vi "WristNetwork_ReadSlow.vi"(8 "error in (no error)":errorcluster) -> (0 "error out":errorcluster)   [LabVIEW 2023]
uses:
  WristGlobal.vi
  <vilib>/Rock Robotics/Network Tables/NT Read Number.vi
  <vilib>/Rock Robotics/Network Tables/NT Read Boolean.vi
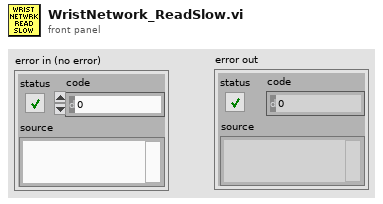
[diagram p1: front panel]
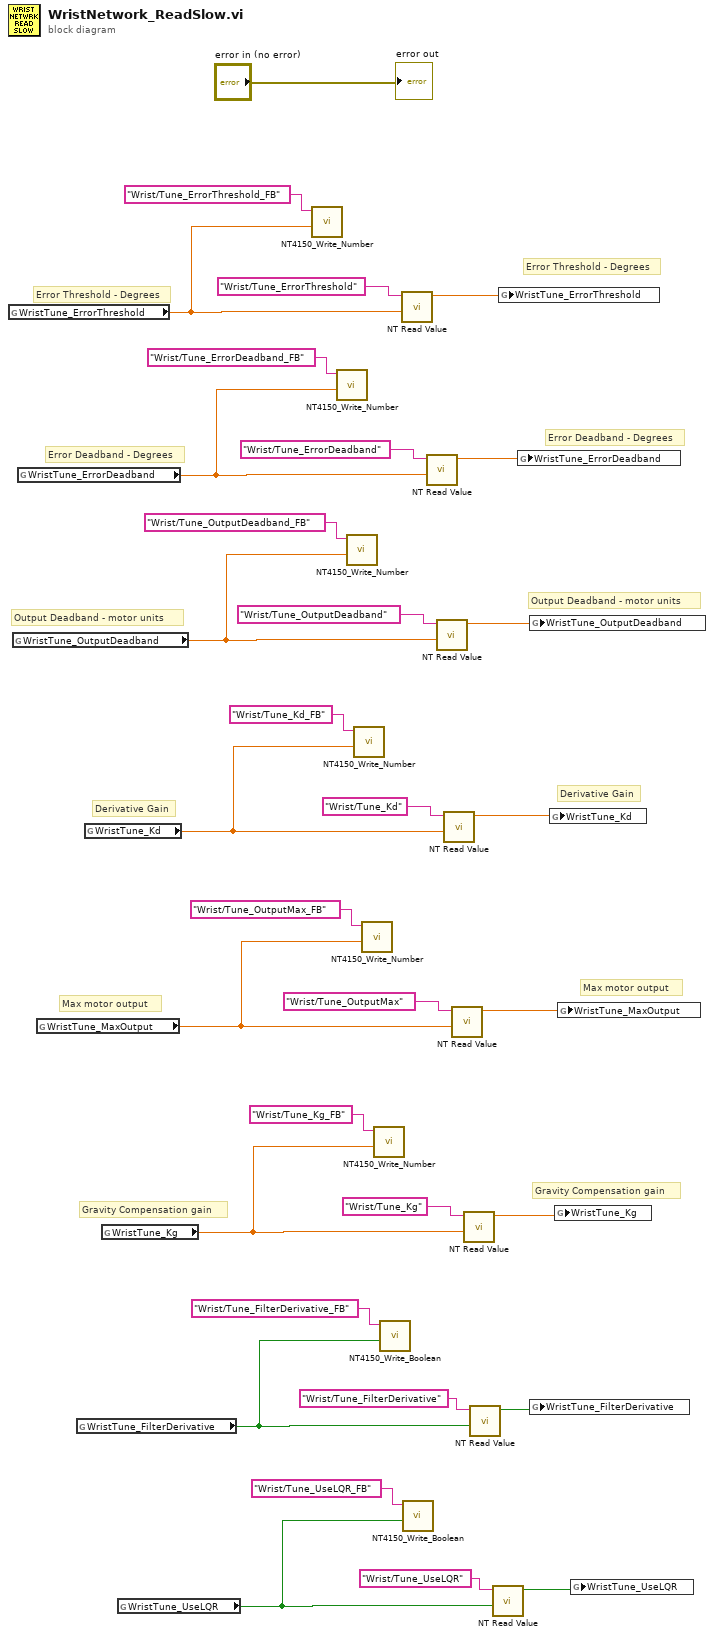
[diagram p0: block diagram]
diagram:
  # "Gravity Compensation gain"
  # "Max motor output"
  # "Derivative Gain"
  # "Output Deadband - motor units"
  # "Error Deadband - Degrees"
  # "Error Threshold - Degrees"
  # "Gravity Compensation gain"
  # "Max motor output"
  # "Derivative Gain"
  # "Output Deadband - motor units"
  # "Error Deadband - Degrees"
  # "Error Threshold - Degrees"
  n1 = global read "WristGlobal.vi" "WristTune_ErrorThreshold"() -> (w30:dbl)
  n2 = global read "WristGlobal.vi" "WristTune_OutputDeadband"() -> (w16:dbl)
  n3 = global read "WristGlobal.vi" "WristTune_ErrorDeadband"() -> (w26:dbl)
  n4 = global read "WristGlobal.vi" "WristTune_MaxOutput"() -> (w12:dbl)
  n5 = global read "WristGlobal.vi" "WristTune_FilterDerivative"() -> (w6:bool)
  n6 = global read "WristGlobal.vi" "WristTune_Kd"() -> (w14:dbl)
  n7 = global read "WristGlobal.vi" "WristTune_Kg"() -> (w10:dbl)
  n8 = global read "WristGlobal.vi" "WristTune_UseLQR"() -> (w2:bool)
  n9 = call "NT4150_Write_Number.vi"("value"=w30, "name"="Wrist/Tune_ErrorThreshold_FB") -> ()  [unwired: 9 in, 1 out]
  n10 = call "NT4150_Write_Number.vi"("value"=w26, "name"="Wrist/Tune_ErrorDeadband_FB") -> ()  [unwired: 9 in, 1 out]
  n11 = call "NT4150_Write_Number.vi"("value"=w16, "name"="Wrist/Tune_OutputDeadband_FB") -> ()  [unwired: 9 in, 1 out]
  n12 = call "NT4150_Write_Number.vi"("value"=w14, "name"="Wrist/Tune_Kd_FB") -> ()  [unwired: 9 in, 1 out]
  n13 = call "NT4150_Write_Number.vi"("value"=w12, "name"="Wrist/Tune_OutputMax_FB") -> ()  [unwired: 9 in, 1 out]
  n14 = call "NT4150_Write_Number.vi"("value"=w10, "name"="Wrist/Tune_Kg_FB") -> ()  [unwired: 9 in, 1 out]
  n15 = call "NT4150_Write_Boolean.vi"("value"=w6, "name"="Wrist/Tune_FilterDerivative_FB") -> ()  [unwired: 9 in, 1 out]
  n16 = call-poly <vilib>:"NT Read Value.vi"("default value"=w30, "name"="Wrist/Tune_ErrorThreshold") -> ("value"=w29:dbl)  [unwired: 7 in, 2 out]
  n17 = call "NT4150_Write_Boolean.vi"("value"=w2, "name"="Wrist/Tune_UseLQR_FB") -> ()  [unwired: 9 in, 1 out]
  n18 = call-poly <vilib>:"NT Read Value.vi"("default value"=w26, "name"="Wrist/Tune_ErrorDeadband") -> ("value"=w25:dbl)  [unwired: 7 in, 2 out]
  n19 = call-poly <vilib>:"NT Read Value.vi"("default value"=w16, "name"="Wrist/Tune_OutputDeadband") -> ("value"=w15:dbl)  [unwired: 7 in, 2 out]
  n20 = call-poly <vilib>:"NT Read Value.vi"("default value"=w14, "name"="Wrist/Tune_Kd") -> ("value"=w13:dbl)  [unwired: 7 in, 2 out]
  n21 = call-poly <vilib>:"NT Read Value.vi"("default value"=w12, "name"="Wrist/Tune_OutputMax") -> ("value"=w11:dbl)  [unwired: 7 in, 2 out]
  n22 = call-poly <vilib>:"NT Read Value.vi"("default value"=w10, "name"="Wrist/Tune_Kg") -> ("value"=w9:dbl)  [unwired: 7 in, 2 out]
  n23 = call-poly <vilib>:"NT Read Value.vi"("default value"=w6, "name"="Wrist/Tune_FilterDerivative") -> ("value"=w5:bool)  [unwired: 7 in, 2 out]
  n24 = call-poly <vilib>:"NT Read Value.vi"("default value"=w2, "name"="Wrist/Tune_UseLQR") -> ("value"=w1:bool)  [unwired: 7 in, 2 out]
  n25 = global write "WristGlobal.vi" "WristTune_ErrorThreshold"(w29) -> ()
  n26 = global write "WristGlobal.vi" "WristTune_ErrorDeadband"(w25) -> ()
  n27 = global write "WristGlobal.vi" "WristTune_OutputDeadband"(w15) -> ()
  n28 = global write "WristGlobal.vi" "WristTune_FilterDerivative"(w5) -> ()
  n29 = global write "WristGlobal.vi" "WristTune_Kd"(w13) -> ()
  n30 = global write "WristGlobal.vi" "WristTune_Kg"(w9) -> ()
  n31 = global write "WristGlobal.vi" "WristTune_MaxOutput"(w11) -> ()
  n32 = global write "WristGlobal.vi" "WristTune_UseLQR"(w1) -> ()
  "error out" <- "error in (no error)"
